vi "ShortcutsTabNameIndex.vi"(8 "OP":T1(ring)=enum."Get", 9 "Enable?":bool=TRUE, 10 "Script":string[][](array[string]), 11 "KeyTabName":string) -> (0 "KeyTableConditionS":string[](array[string]), 1 "Enable?S":bool[](array[boolean]), 2 "Scripts":cluster{"Script":string[][]}[](array[cluster]), 3 "KeyTabNameS":string[](array[string]))   [LabVIEW 2020]
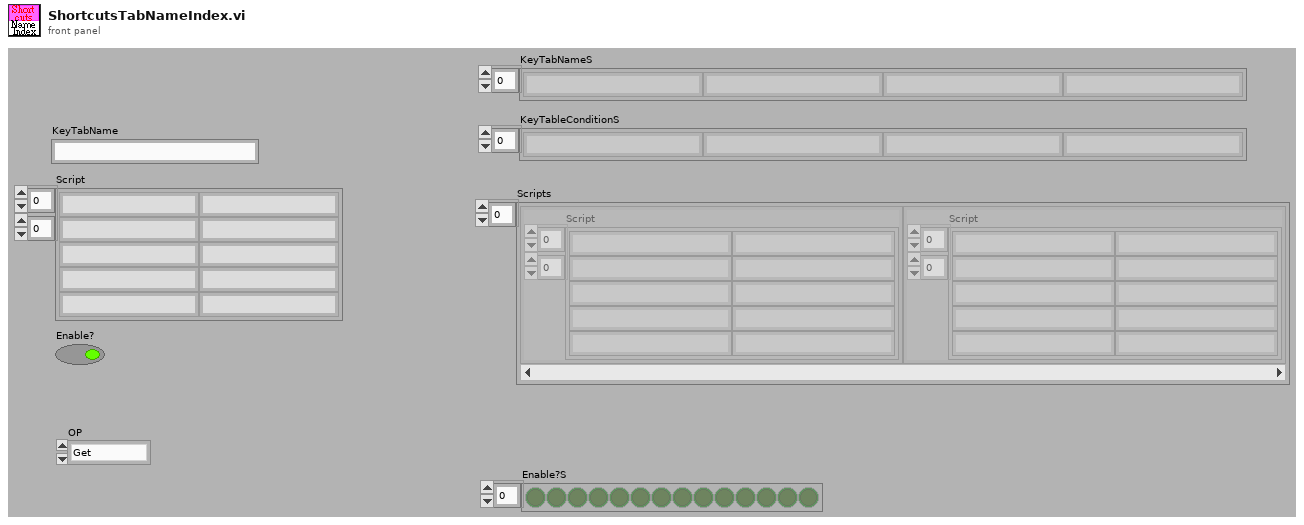
[diagram p1: front panel]
types:
  T1 = enum16{"Init", "Add", "Enable", "Disable", "Get"}
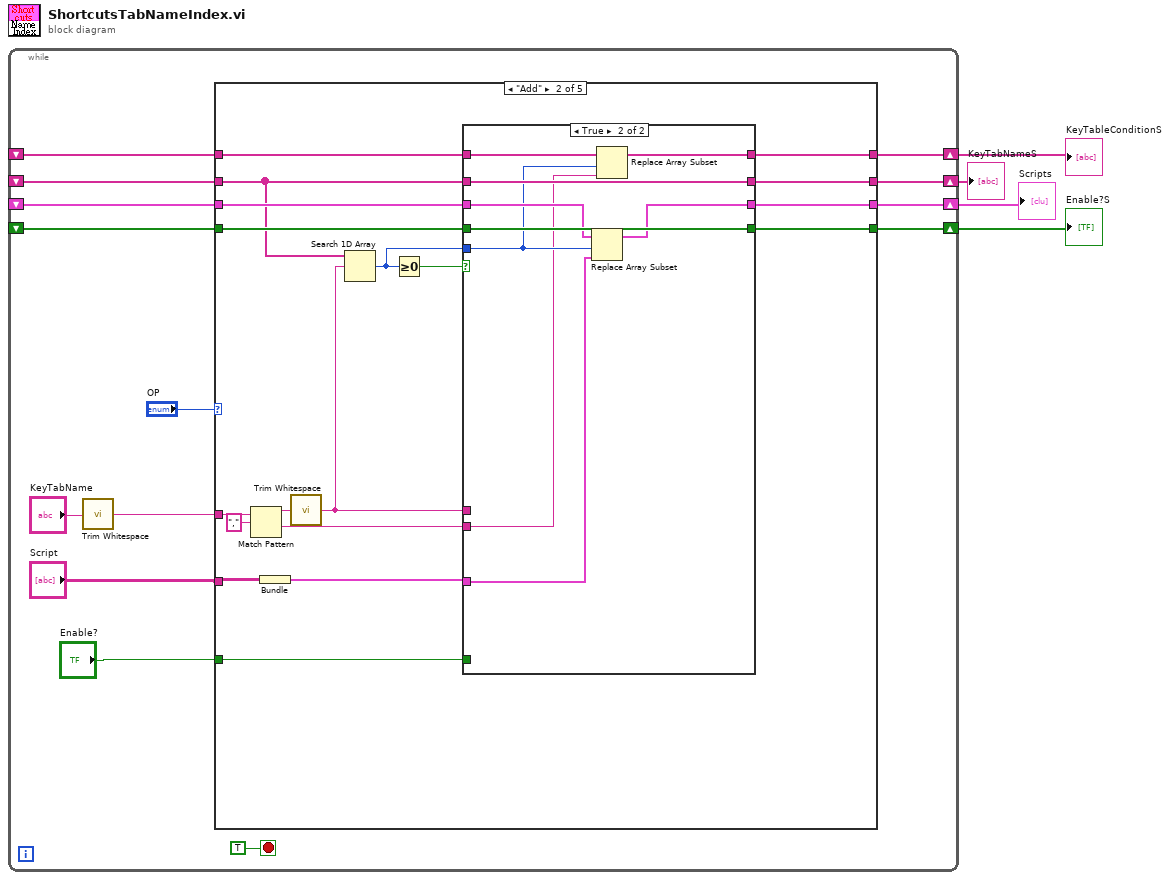
[diagram p0: block diagram]
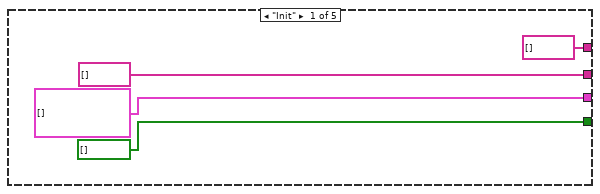
[diagram p2: hidden frame]
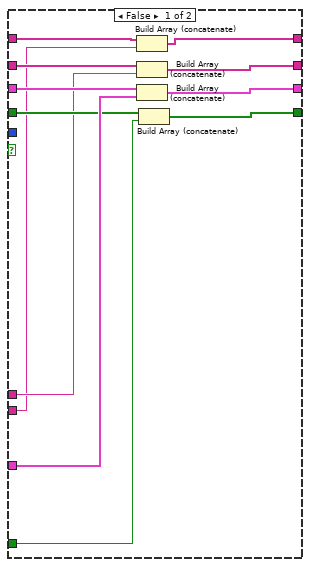
[diagram p3: hidden frame]
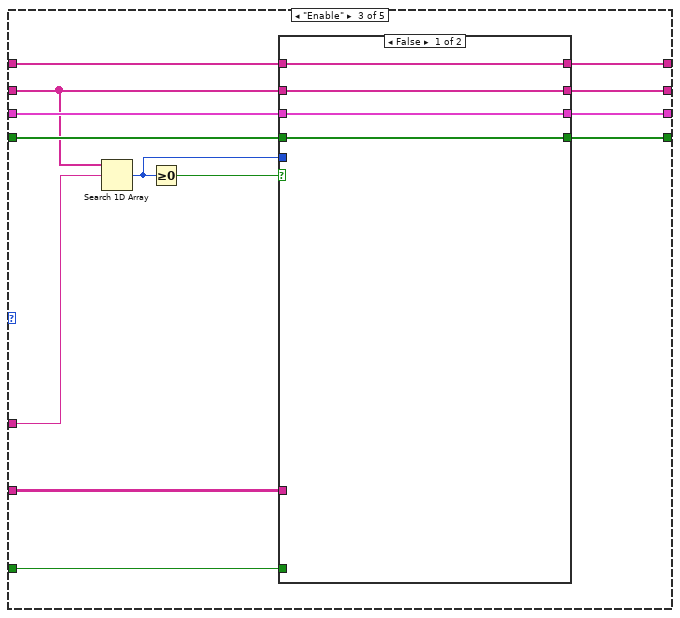
[diagram p4: hidden frame]
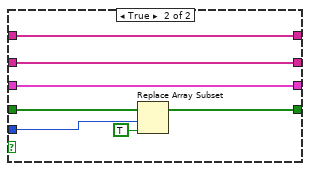
[diagram p5: hidden frame]
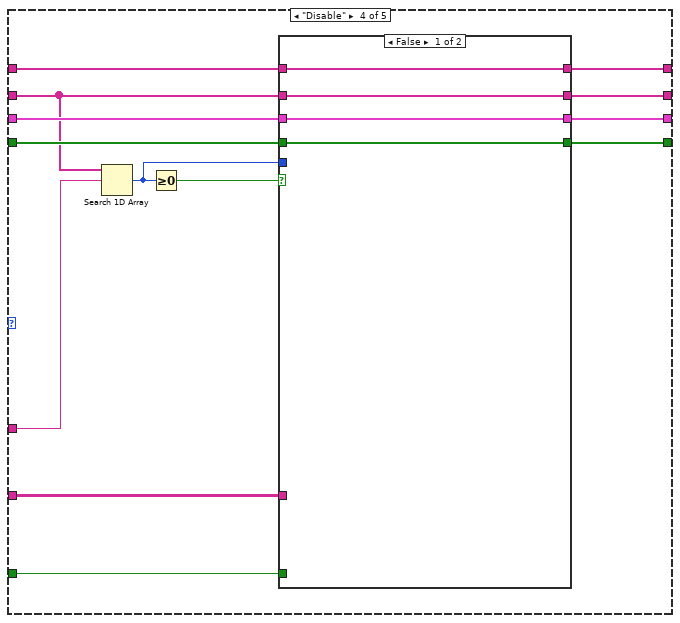
[diagram p6: hidden frame]
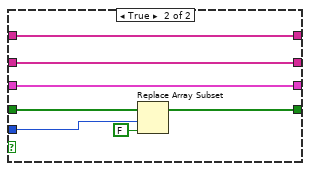
[diagram p7: hidden frame]
diagram:
  n1 = while {
    shift-right: [w16] -> w3
    shift-left: _ -> [w15]
    shift-right: [w14] -> w2
    shift-left: _ -> [w13]
    shift-right: [w10] -> w4
    shift-left: _ -> [w9]
    shift-right: [w6] -> w1
    shift-left: _ -> [w5]
    stop <- TRUE stop-if-true
    n2 = call <vilib>:"Trim Whitespace.vi"("string"="KeyTabName") -> ("trimmed string"=w11:string)  [unwired: 1 in]
    n3 = case shown="\"Add\"" "OP" {
      tunnel: "Script" -> [_ w31 w74 w98 _]
      tunnel: "Enable?" -> [_ w35 w68 w92 _]
      tunnel: [cluster{"Script":string[][]}[] [] w39 w72 w96 w112] -> w16
      tunnel: w15 -> [_ w40 w73 w97 w112]
      tunnel: [bool[] [] w38 w71 w95 w111] -> w14
      tunnel: w13 -> [_ w37 w70 w94 w111]
      tunnel: w11 -> [_ w29 w66 w90 _]
      tunnel: [string[] [] w36 w69 w93 w113] -> w10
      tunnel: w9 -> [_ w34 w67 w91 w113]
      tunnel: [string[] [] w26 w62 w86 w110] -> w6
      tunnel: w5 -> [_ w25 w63 w87 w110]
      frame "Init" {
      }
      frame "Add" {
        n4 = Match Pattern(string=w29, regular expression=",") -> (before substring=w24:string, after substring=w27:string)  [unwired: 1 in, 2 out]
        n5 = Bundle("Script"=w31) -> (w30:cluster{"Script":string[][]})  [unwired: 1 in]
        n6 = call <vilib>:"Trim Whitespace.vi"("string"=w24) -> ("trimmed string"=w23:string)  [unwired: 1 in]
        n7 = Search 1D Array(1D array=w34, element=w23) -> (index of element=w32:i32)  [unwired: 1 in]
        n8 = Greater Or Equal To 0?(x=w32) -> (x >= 0?=w33:bool)
        n9 = case shown="True" w33 {
          tunnel: w30 -> [w52 w58]
          tunnel: w40 -> [w51 w59]
          tunnel: [w50 w57] -> w39
          tunnel: [w49 w60] -> w38
          tunnel: w37 -> [w48 w60]
          tunnel: [w47 w61] -> w36
          tunnel: w34 -> [w46 w61]
          tunnel: w35 -> [w45 _]
          tunnel: w32 -> [_ w55]
          tunnel: w23 -> [w44 _]
          tunnel: w27 -> [w43 w53]
          tunnel: [w42 w54] -> w26
          tunnel: w25 -> [w41 w56]
          frame False {
            n10 = Build Array (concatenate)(w41, w43) -> (w42:string[])
            n11 = Build Array (concatenate)(w46, w44) -> (w47:string[])
            n12 = Build Array (concatenate)(w51, w52) -> (w50:cluster{"Script":string[][]}[])
            n13 = Build Array (concatenate)(w48, w45) -> (w49:bool[])
          }
          frame True {
            n14 = Replace Array Subset(array=w59, new element=w58, index=w55) -> (w57:cluster{"Script":string[][]}[])
            n15 = Replace Array Subset(array=w56, new element=w53, index=w55) -> (w54:string[])
          }
        }
      }
      frame "Enable" {
        n16 = Search 1D Array(1D array=w67, element=w66) -> (index of element=w64:i32)  [unwired: 1 in]
        n17 = Greater Or Equal To 0?(x=w64) -> (x >= 0?=w65:bool)
        n18 = case shown="False" w65 {
          tunnel: w74 -> [_ _]
          tunnel: w73 -> [w77 w83]
          tunnel: [w77 w83] -> w72
          tunnel: [w76 w81] -> w71
          tunnel: w70 -> [w76 w82]
          tunnel: [w78 w85] -> w69
          tunnel: w67 -> [w78 w85]
          tunnel: w68 -> [_ _]
          tunnel: w64 -> [_ w84]
          tunnel: w63 -> [w75 w79]
          tunnel: [w75 w79] -> w62
          frame False {
          }
          frame True {
            n19 = Replace Array Subset(array=w82, new element=TRUE ("new element/subarray"), index=w84) -> (w81:bool[])
          }
        }
      }
      frame "Disable" {
        n20 = Search 1D Array(1D array=w91, element=w90) -> (index of element=w88:i32)  [unwired: 1 in]
        n21 = Greater Or Equal To 0?(x=w88) -> (x >= 0?=w89:bool)
        n22 = case shown="False" w89 {
          tunnel: w98 -> [_ _]
          tunnel: w97 -> [w101 w107]
          tunnel: [w101 w107] -> w96
          tunnel: [w100 w105] -> w95
          tunnel: w94 -> [w100 w106]
          tunnel: [w102 w109] -> w93
          tunnel: w91 -> [w102 w109]
          tunnel: w92 -> [_ _]
          tunnel: w88 -> [_ w108]
          tunnel: w87 -> [w99 w103]
          tunnel: [w99 w103] -> w86
          frame False {
          }
          frame True {
            n23 = Replace Array Subset(array=w106, new element=FALSE ("new element/subarray"), index=w108) -> (w105:bool[])
          }
        }
      }
      frame "Get" {
      }
    }
  }
  "KeyTabNameS" <- w4
  "Scripts" <- w3
  "Enable?S" <- w2
  "KeyTableConditionS" <- w1
